vi "Xylo_Essai_1.vi"   [LabVIEW 2018]
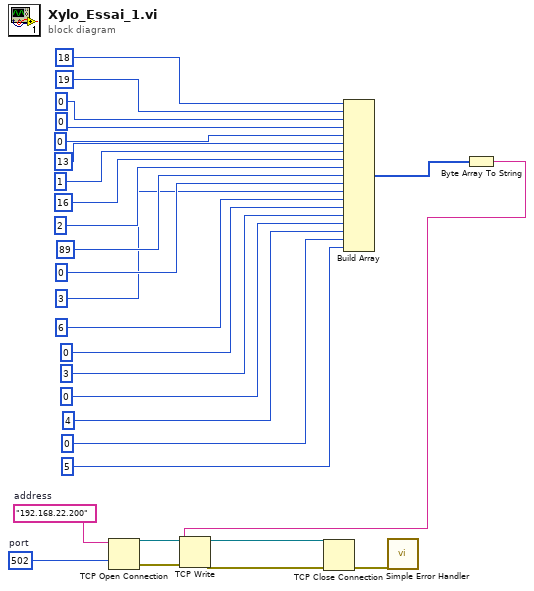
[diagram p0: block diagram]
diagram:
  w28 = "192.168.22.200"  # address
  w27 = 502  # port
  n1 = TCP Open Connection(address=w28, remote port or service name=w27) -> (connection ID=w9:refnum<k5>, error out=w10:errorcluster)  [unwired: 3 in]
  n2 = Build Array(18, 19, 0, 0, 0, 13, 1, 16, 2, 89, 0, 3 ("element"), 6, 0, 3, 0, 4, 0, 5 ("element")) -> (w23:i32[])
  n3 = Byte Array To String(unsigned byte array=w23) -> (string=w25:string)
  n4 = TCP Write(connection ID=w9, data in=w25, error in (no error)=w10) -> (connection ID out=w22:refnum<k5>, error out=w21:errorcluster)  [unwired: 1 in, 1 out]
  n5 = TCP Close Connection(connection ID=w22, error in (no error)=w21) -> (error out=w26:errorcluster)  [unwired: 1 in, 1 out]
  n6 = call <vilib>:"Simple Error Handler.vi"("error in (no error)"=w26) -> ()  [unwired: 4 in, 5 out]
